vi "ws_edittest parse query params.vi"(11 "httpRequestID":u32) -> (0 "Client Address":string, 1 "First Value":string, 2 "First Key":string, 3 "Query Parameters":T1)   [LabVIEW 2011]
uses:
  <vilib>/addons/internet/utils/keyedarr.llb/Keyed Array.ctl
  <vilib>/addons/internet/utils/strutil.llb/Case Matching.ctl
  <vilib>/wsapi/NI_WebServices.lvlib
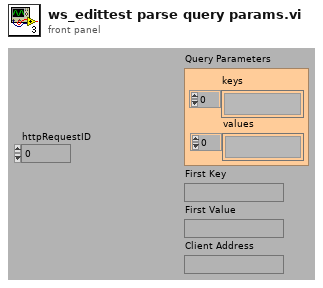
[diagram p1: front panel]
types:
  T1 = typedef "Keyed Array.ctl" = cluster{"keys":string[], "values":string[]}
  T2 = typedef "Case Matching.ctl" = enum16{"a != A", "a == A", "system"}
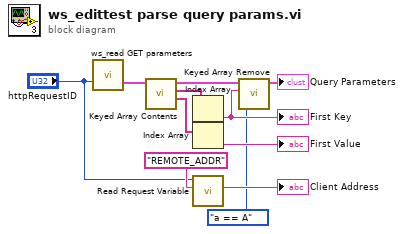
[diagram p0: block diagram]
diagram:
  n1 = call "ws_read GET parameters.vi"("httpRequestID"="httpRequestID") -> ("GET query params"=w2:T1)  [unwired: 2 in]
  n2 = call <vilib>:"Keyed Array Contents.vi"("array in"=w2) -> ("values"=w8:string[], "keys"=w11:string[], "duplicate array"=w10:T1)  [unwired: 4 in]
  n3 = Index Array(array=w11) -> (element=w7:string)  [unwired: 1 in]
  "First Key" <- w7
  n4 = Index Array(array=w8) -> (element=→"First Value":string)  [unwired: 1 in]
  n5 = call <vilib>:"Read Request Variable.vi"("variable name"="REMOTE_ADDR" ("key"), "httpRequestID"="httpRequestID") -> ("value"=→"Client Address":string)  [unwired: 7 in, 2 out]
  n6 = call <vilib>:"Keyed Array Remove.vi"("case matching (sensitive)"=Case_Matching."a == A", "key"=w7, "array in"=w10) -> ("array out"=→"Query Parameters":T1)  [unwired: 2 in, 2 out]
